vi "Sinc Pattern.vi"(2 "delta t":dbl=0.1 format="%0.2f", 3 "delay":dbl format="%0.2f", 4 "amplitude":dbl=1.0 format="%0.2f", 5 "samples":i32=128) -> (0 "error":i32, 1 "Sinc Pattern":dbl[](array[numeric]))   [LabVIEW 2010, in "NI_AALBase.lvlib"]
doc: "Generates an array containing a sinc pattern."
uses:
  NI_AALBase.lvlib
  lvanlys.dll
panel:
  # "Sinc Pattern"
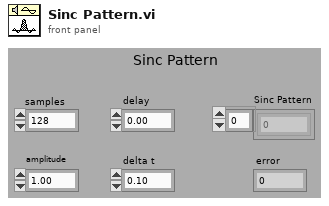
[diagram p1: front panel]
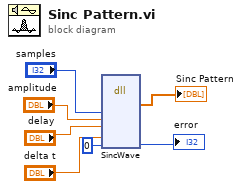
[diagram p0: block diagram]
diagram:
  n1 = dll-call lib="C:/Program Files/National Instruments/LabVIEW 2010/resource/lvanlys.*" fn="SincWave"("samples"="samples", "amplitude"="amplitude", "delay"="delay", "delta t"="delta t", 0) -> ("Sinc Pattern"=→"Sinc Pattern":dbl[], →"error":i32)  [unwired: 9 in, 2 out]
